vi "test_labview.vi"() -> ()   [LabVIEW 2016]
panel:
  out "status code":dbl=4353.0
  out "array":dbl[][](array[numeric])=[[1.0, 21745730.0, 4353.0]]
  out "XY Graph":cluster{dbl[], dbl[]}(graph)={[100.0, 90.0, 80.0, 70.0, 60.0, 50.0, 40.0, 30.0, 20.0, 10.0, 0.0, -10.0, -20.0], [0.000776771, 0.00077701, 0.000776831, 0.000777368, 0.00077701, 0.000777069, 0.000776354, 0.000776831, 0.00077695, 0.00077701, 0.000776593, 0.000776473, 0.000776533, 0.000777368, 0.000776712, 0.000777069, 0.000776712, 0.000776831, 0.00077695, 0.000776414, 0.00077701, 0.000776712, 0.000777189, 0.000776831, 0.000776712, 0.000776771, 0.000777189, 0.000776533, 0.000776295, 0.000776473, 0.000776771, 0.00077695, 0.000776831]}
  out "number":dbl=0.000776831
  in  "SR830 GPIB Addr":string="9"
  in  "Temp":dbl=300.0
  in  "Num of pts":dbl=20.0
  in  "Max Field":dbl=100.0
  in  "PPMS GPIB Addr":string="15"
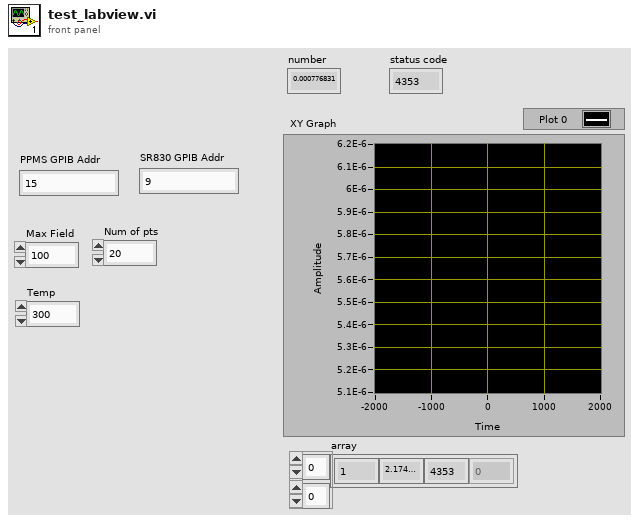
[diagram p1: front panel]
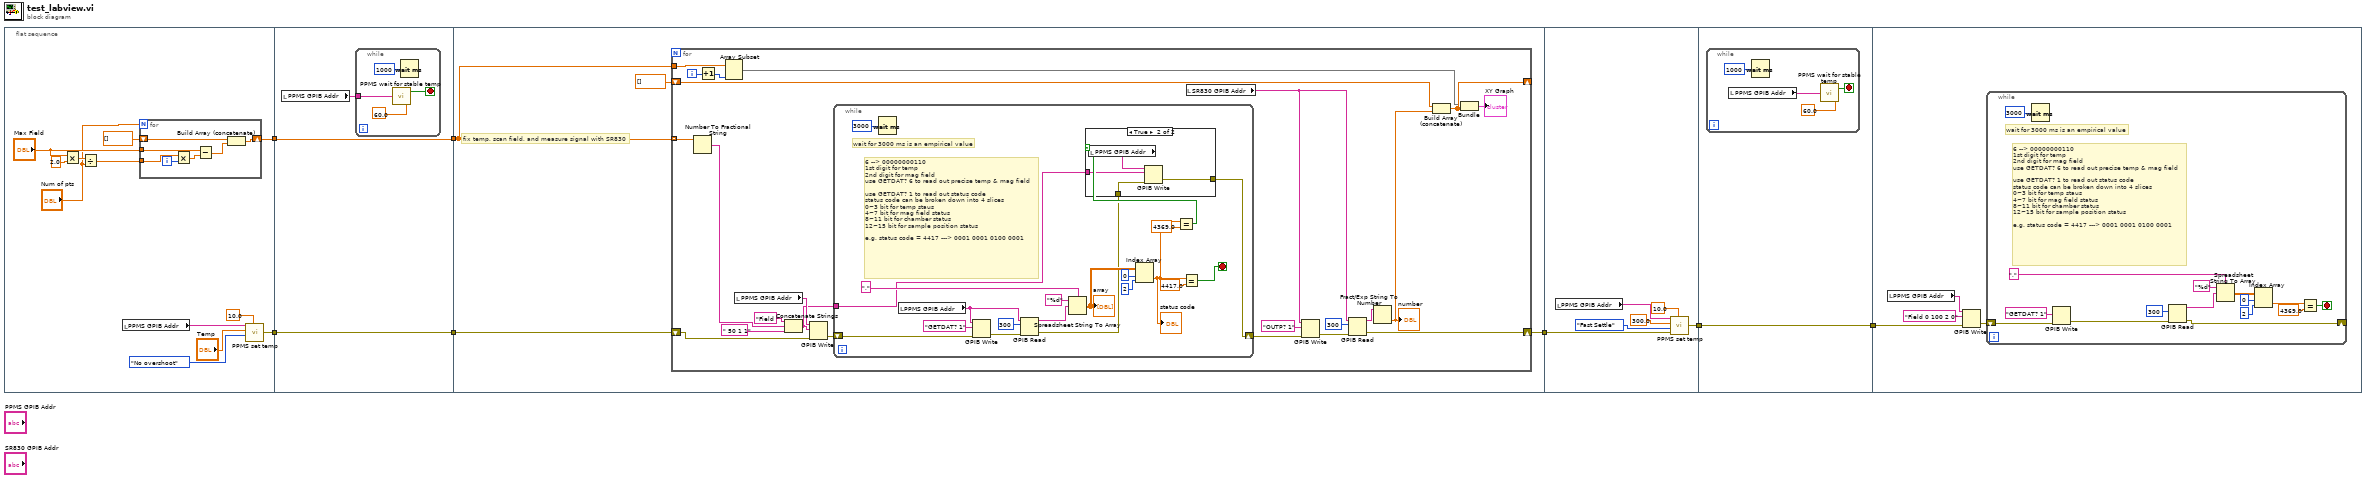
[diagram p0: block diagram]
diagram:
  n1 = flat-sequence {
    tunnel: [w9] -> w7
    tunnel: [w8] -> w5
    tunnel: w7 -> [w29]
    tunnel: [w29] -> w6
    tunnel: w5 -> [w28]
    tunnel: [w28] -> w4
    tunnel: w6 -> [w36]
    tunnel: w4 -> [w37]
    tunnel: [w34] -> w3
    tunnel: w3 -> [w88]
    tunnel: [w87] -> w2
    tunnel: w2 -> [w92]
    tunnel: [w92] -> w1
    tunnel: w1 -> [w98]
    frame #0 {
      n2 = Multiply(x="Max Field", y=2.0) -> (x*y=w14:dbl)
      n3 = Divide(x=w14, y="Num of pts") -> (x/y=w12:dbl)
      n4 = local read "PPMS GPIB Addr"() -> (w16:string)
      n5 = for {
        N: "Num of pts" -> [_]
        shift-right: [w21] -> w9
        shift-left: dbl[] [] -> [w20]
        tunnel: "Max Field" -> [w26]
        tunnel: w12 -> [w24]
        i -> [w25]
        n6 = Multiply(x=w24, y=w25) -> (x*y=w23:dbl)
        n7 = Subtract(x=w26, y=w23) -> (x-y=w22:dbl)
        n8 = Build Array (concatenate)(w20, w22) -> (w21:dbl[])
      }
      n9 = call "PPMS set temp.vi"("PPMS GPIB address"=w16, "Set Temperature"="Temp", "Approach Method"=enum16{"Fast Settle", "No overshoot"}."No overshoot", "Approach Rate( 0-20)"=10.0) -> ("error out"=w8:errorcluster)  [unwired: 1 in]
    }
    frame #1 {
      n10 = local read "PPMS GPIB Addr"() -> (w27:string)
      n11 = while {
        tunnel: w27 -> [w33]
        stop <- w32 stop-if-true
        n12 = call "PPMS wait for stable temp.vi"("Wait for (s)"=60.0, "GPIB address"=w33) -> ("Temperature Stabilized?"=w32:bool)  [unwired: 2 in]
        n13 = Wait (ms)(milliseconds to wait=u32 1000) -> ()  [unwired: 1 out]
      }
    }
    frame #2 {
      # "fix temp, scan field, and measure signal with SR830"
      n14 = for {
        tunnel: w36 -> [w42] mode=indexing
        shift-right: [w55] -> w34
        shift-left: w37 -> [w44]
        shift-right: [w49] -> _
        shift-left: dbl[] [] -> [w53]
        tunnel: w36 -> [w52]
        i -> [w51]
        n15 = Number To Fractional String(number=w42) -> (F-format string=w40:string)  [unwired: 3 in]
        n16 = Increment(x=w51) -> (x+1=w50:i32)
        n17 = Array Subset(array=w52, length=w50) -> (w48:dbl[])  [unwired: 1 in]
        n18 = local read "PPMS GPIB Addr"() -> (w45:string)
        n19 = Concatenate Strings("Field " ("string"), w40, " 50 1 1" ("string")) -> (w38:string)
        n20 = GPIB Write(0:w45, 1:w38, 3:w44) -> (6:w43:errorcluster)  [unwired: 2 in, 1 out]
        n21 = while {
          shift-right: [w61] -> w46
          shift-left: w43 -> [w69]
          tunnel: w38 -> [w63]
          stop <- w67 stop-if-true
          # "wait for 3000 ms is an empirical value"
          # "6 --> 00000000110\n1st digit for temp\n2nd digit for mag field\nuse GETDAT? 6 to read out precise temp & mag field\n\nuse GETDAT? 1 to read out status code\nstatus code can be broken down into 4 slices\n0~3 bit for temp staus\n4~7 bit for mag field status\n8~11 bit for chamber status\n12~15 bit for sample position status\n\ne.g. status code = 4417 ---> 0001 0001 0100 0001"
          n22 = Wait (ms)(milliseconds to wait=u32 3000) -> ()  [unwired: 1 out]
          n23 = local read "PPMS GPIB Addr"() -> (w78:string)
          n24 = GPIB Write(0:w78, 1:"GETDAT? 1" ("data"), 3:w69) -> (6:w77:errorcluster)  [unwired: 2 in, 1 out]
          n25 = GPIB Read(0:w78, 1:300 ("byte count"), 3:w77) -> (5:w74:string, 7:w62:errorcluster)  [unwired: 2 in, 1 out]
          n26 = Spreadsheet String To Array(delimiter (Tab)=",", format string="%d", spreadsheet string=w74) -> (array=w73:dbl[][])  [unwired: 1 in]
          "array" <- w73
          n27 = Index Array(array=w73, index (row)=0, index (col)=2 ("disabled index (col)")) -> (element=w66:dbl)
          "status code" <- w66
          n28 = Equal?(x=w66, y=4369.0) -> (x = y?=w64:bool)
          n29 = case shown="True" w64 {
            tunnel: w63 -> [_ w84]
            tunnel: w62 -> [w81 w83]
            tunnel: [w81 w82] -> w61
            frame False {
            }
            frame True {
              n30 = local read "PPMS GPIB Addr"() -> (w85:string)
              n31 = GPIB Write(0:w85, 1:w84, 3:w83) -> (6:w82:errorcluster)  [unwired: 2 in, 1 out]
            }
          }
          n32 = Equal?(x=w66, y=4417.0) -> (x = y?=w67:bool)
        }
        n33 = local read "SR830 GPIB Addr"() -> (w58:string)
        n34 = GPIB Write(0:w58, 1:"OUTP? 1" ("data"), 3:w46) -> (6:w60:errorcluster)  [unwired: 2 in, 1 out]
        n35 = GPIB Read(0:w58, 1:300 ("byte count"), 3:w60) -> (5:w56:string, 7:w55:errorcluster)  [unwired: 2 in, 1 out]
        n36 = Fract/Exp String To Number(string=w56) -> (number=w54:dbl)  [unwired: 3 in, 1 out]
        "number" <- w54
        n37 = Build Array (concatenate)(w53, w54) -> (w49:dbl[])
        n38 = Bundle(w48, w49) -> (→"XY Graph":cluster{dbl[], dbl[]})  [unwired: 1 in]
      }
    }
    frame #3 {
      n39 = local read "PPMS GPIB Addr"() -> (w86:string)
      n40 = call "PPMS set temp.vi"("PPMS GPIB address"=w86, "Set Temperature"=300.0, "Approach Method"=enum16{"Fast Settle", "No overshoot"}."Fast Settle", "error in (no error)"=w88, "Approach Rate( 0-20)"=10.0) -> ("error out"=w87:errorcluster)
    }
    frame #4 {
      n41 = while {
        stop <- w96 stop-if-true
        n42 = local read "PPMS GPIB Addr"() -> (w93:string)
        n43 = Wait (ms)(milliseconds to wait=u32 1000) -> ()  [unwired: 1 out]
        n44 = call "PPMS wait for stable temp.vi"("Wait for (s)"=60.0, "GPIB address"=w93) -> ("Temperature Stabilized?"=w96:bool)  [unwired: 2 in]
      }
    }
    frame #5 {
      n45 = local read "PPMS GPIB Addr"() -> (w100:string)
      n46 = GPIB Write(0:w100, 1:"Field 0 100 2 0" ("data"), 3:w98) -> (6:w99:errorcluster)  [unwired: 2 in, 1 out]
      n47 = while {
        shift-right: [w109] -> _
        shift-left: w99 -> [w102]
        stop <- w105 stop-if-true
        # "wait for 3000 ms is an empirical value"
        # "6 --> 00000000110\n1st digit for temp\n2nd digit for mag field\nuse GETDAT? 6 to read out precise temp & mag field\n\nuse GETDAT? 1 to read out status code\nstatus code can be broken down into 4 slices\n0~3 bit for temp staus\n4~7 bit for mag field status\n8~11 bit for chamber status\n12~15 bit for sample position status\n\ne.g. status code = 4417 ---> 0001 0001 0100 0001"
        n48 = Wait (ms)(milliseconds to wait=u32 3000) -> ()  [unwired: 1 out]
        n49 = GPIB Write(1:"GETDAT? 1" ("data"), 3:w102) -> (6:w113:errorcluster)  [unwired: 3 in, 1 out]
        n50 = GPIB Read(1:300 ("byte count"), 3:w113) -> (5:w110:string, 7:w109:errorcluster)  [unwired: 3 in, 1 out]
        n51 = Spreadsheet String To Array(delimiter (Tab)=",", format string="%d", spreadsheet string=w110) -> (array=w108:dbl[][])  [unwired: 1 in]
        n52 = Index Array(array=w108, index (row)=0, index (col)=2 ("disabled index (col)")) -> (element=w103:dbl)
        n53 = Equal?(x=w103, y=4369.0) -> (x = y?=w105:bool)
      }
    }
  }
